vi "Tools VIs.vi"(6 "IMAQ Image Display Ref":refnum<vi>, 8 "Tool Name Text Ref":refnum<vi>, 9 "Left (Screen Coords, px)":i32=50, 11 "Top (Screen Coords, px)":i32=50) -> ()   [LabVIEW 2016]
uses:
  <vilib>/Utility/miscctls.llb/LVPointTypeDef.ctl
  <vilib>/Utility/miscctls.llb/LVRectTypeDef.ctl
  User32.dll
panel:
  in  "Show Cursor":bool=TRUE
  in  "Tools and ROI Menu":T1(radio)
  in  "Color Map Menu":T2(radio)
  in  "Scale All to This":bool
  in  "Load Image":bool
  in  "Tools and ROIs":bool
  in  "Lock Zoom and Pan Tools":bool
  in  "Pan Tool":bool
  in  "Reset Zoom":bool
  in  "Zoom Out":bool
  in  "Zoom In":bool
  in  "Auto Scale All":bool
  in  "Auto Scale":bool
  in  "Color Map":bool
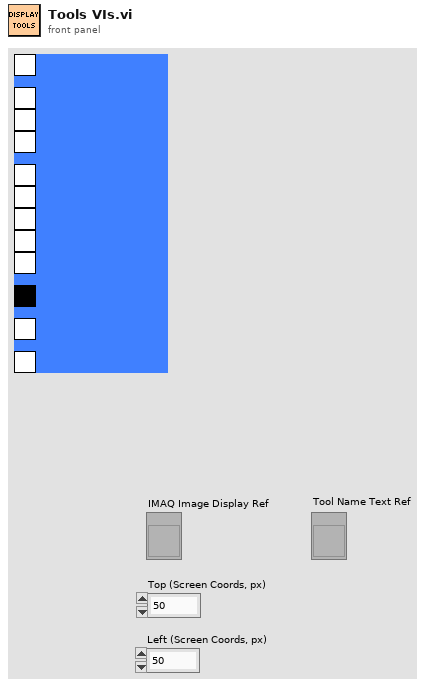
[diagram p1: front panel]
types:
  T1 = enum32{"Fitting Tool", "Merge Tool", "Smooth Tool", "Rectangular ROI", "Free Form ROI", "Clear ROI"}
  T2 = enum32{"Blue Z Scale", "Blue-White Z Scale", "Cyan Z Scale", "Fire Z Scale", "Glow Z Scale", "Green", "Green-White Z Scale", "Magenta Z Scale", "Red Z Scale", "Red-White Z Scale", "Yellow Z Scale"}
  T3 = enum32{"Invalid", "Standard", "Closed", "Hidden", "Minimized", "Maximized"}
  T4 = typedef "LVRectTypeDef.ctl" = cluster{"Left":i16, "Top":i16, "Right":i16, "Bottom":i16}
  T5 = typedef "LVPointTypeDef.ctl" = cluster{"Horizontal":i16, "Vertical":i16}
  T6 = enum16{"Always On", "Always Off", "Off While Running"}
  T7 = enum32{"Bad", "Idle", "Run top level", "Running"}
  T8 = typedef "lveventtype.ctl" = enum32{"Null", "Timeout", "Annotation Menu Selection", "Annotation Menu Selection?", "App Instance Close", "App Instance Close?", "Autoscale Range Change", "Bookmark Info Change", "Cell Edit", "Cell Edit?", "Cursor Grab", "Cursor Grab?", "Cursor Menu Selection", "Cursor Menu Selection?", "Cursor Move", "Cursor Release", "Data Change", "Direction Change", "Display State Change", "Drag Ended", "Drag Enter", "Drag Leave", "Drag Over", "Drag Source Update", "Drag Starting", "Drag Starting?", "Drop", "Exec State Change", "Key Down", "Key Down?", "Key Repeat", "Key Repeat?", "Key Up", "Listbox Double Click", "Menu Activation?", "Menu Selection (App)", "Menu Selection? (App)", "Menu Selection (User)", "Mouse Down", "Mouse Down?", "Mouse Enter", "Mouse Leave", "Mouse Move", "Mouse Up", "Mouse Wheel", "NI Security User Change (App)", "Pane Size", "Panel Close", "Panel Close?", "Panel Resize", "Plot Attribute Change", "Scale Range Change", "Shortcut Menu Activation?", "Shortcut Menu Selection (App)", "Shortcut Menu Selection? (App)", "Shortcut Menu Selection (User)", "Tree Double Click", "Tree Drag", "Tree Drag?", "Tree Drop", "Tree Drop?", "Tree Item Close", "Tree Item Close?", "Tree Item Open", "Tree Item Open?", "User Event", "Value Change"}
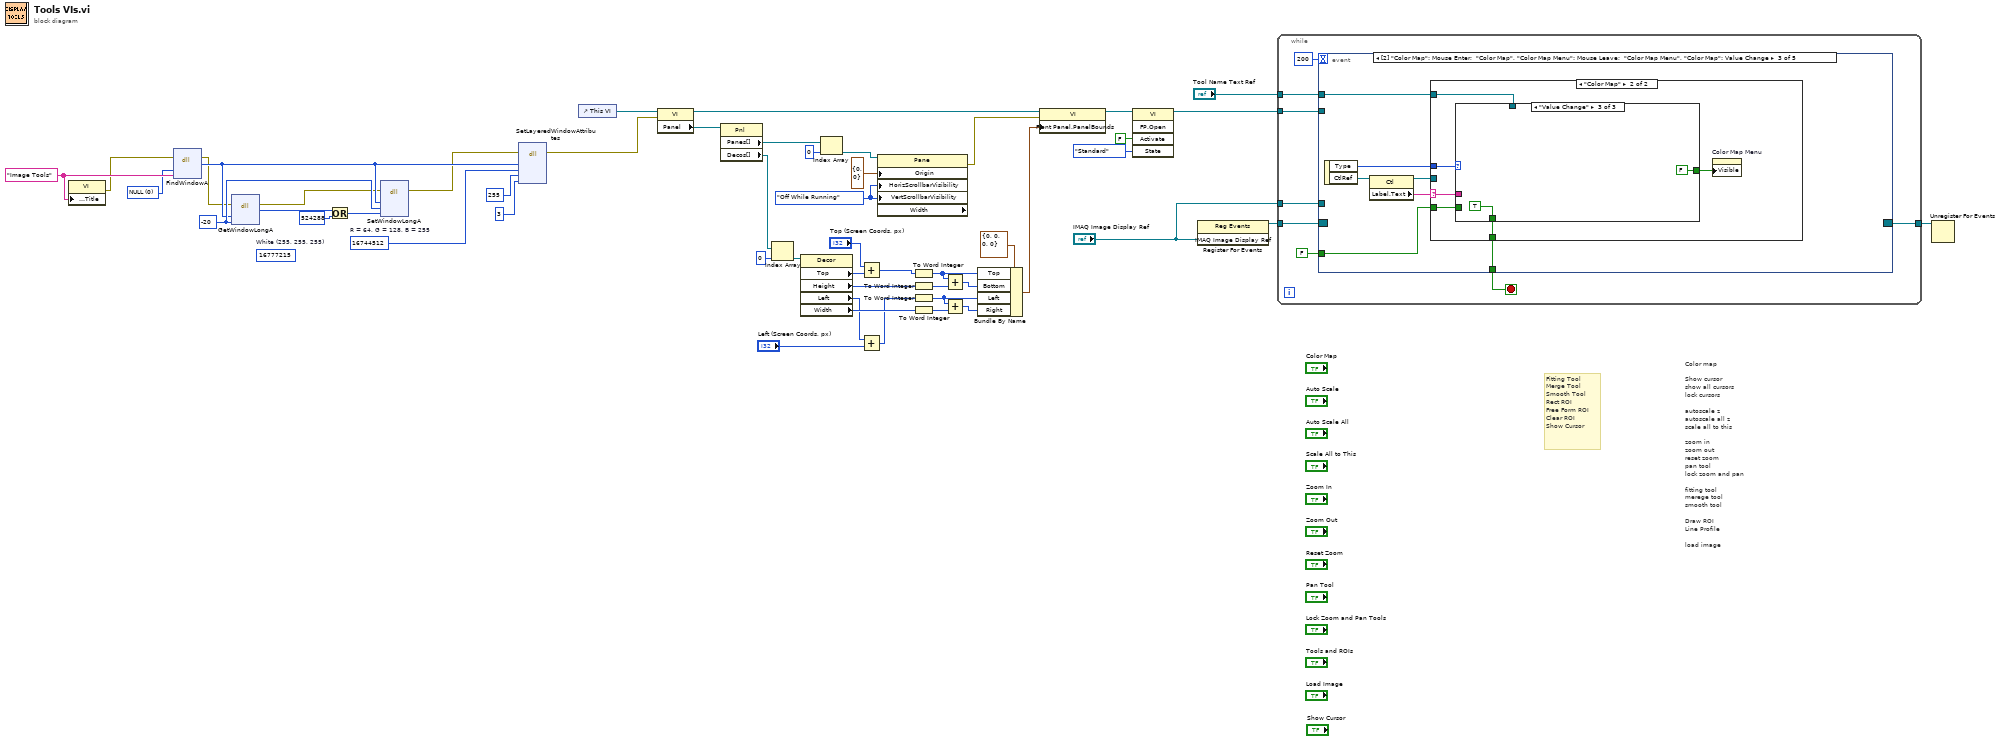
[diagram p0: block diagram]
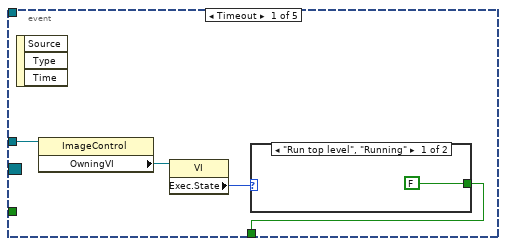
[diagram p2: hidden frame]
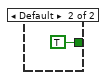
[diagram p3: hidden frame]
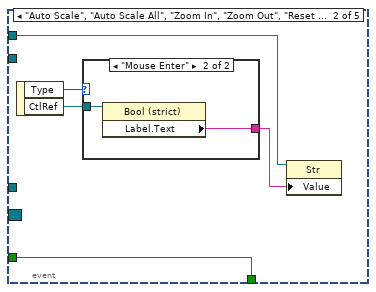
[diagram p4: hidden frame]
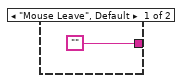
[diagram p5: hidden frame]
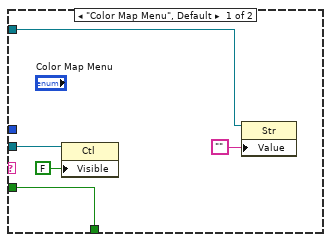
[diagram p6: hidden frame]
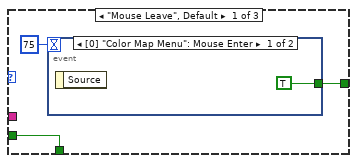
[diagram p7: hidden frame]
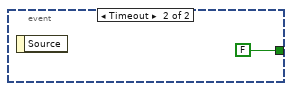
[diagram p8: hidden frame]
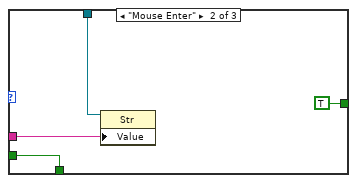
[diagram p9: hidden frame]
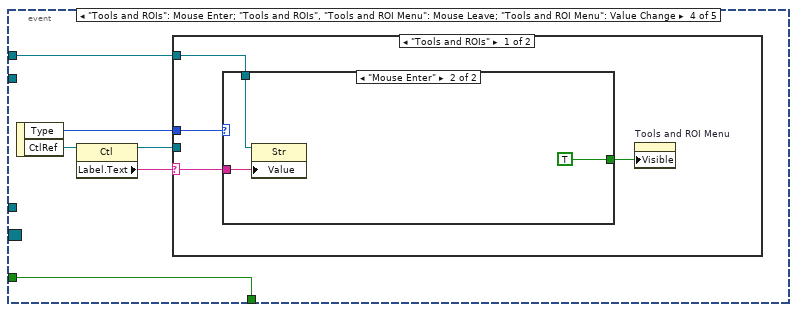
[diagram p10: hidden frame]
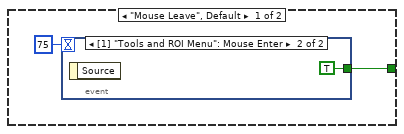
[diagram p11: hidden frame]
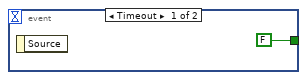
[diagram p12: hidden frame]
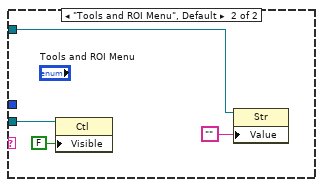
[diagram p13: hidden frame]
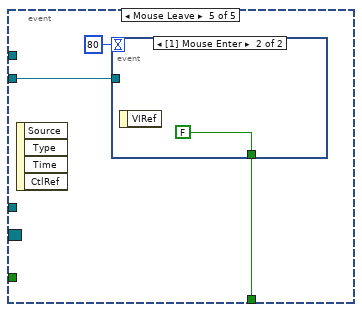
[diagram p14: hidden frame]
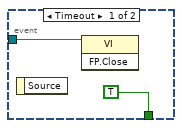
[diagram p15: hidden frame]
diagram:
  w11 = 16744512  # R = 64, G = 128, B = 255
  (unwired) 16777215  # White (255, 255, 255)
  w17 = 0 items=["NULL"]
  w21 = -20 ("nIndex")
  w23 = "Image Tools" ("Front Panel Window:Title")
  w47 = T6."Off While Running" ("Horizontal Scrollbar Visibility")
  # "Fitting Tool\nMerge Tool\nSmooth Tool\nRect ROI\nFree Form ROI\nClear ROI\nShow Cursor"
  # "Color map\n\nShow cursor\nshow all cursors\nlock cursors\n\nautoscale z\nautoscale all z\nscale all to this\n\nzoom in\nzoom out\nreset zoom\npan tool\nlock zoom and pan\n\nfitting tool\nmerege tool\nsmooth tool\n\nDraw ROI\nLine Profile\n\nload image"
  n1 = property class="VI"("Front Panel.Title"=w23) -> (error out=w10:errorcluster)  [unwired: 2 in, 1 out]
  n2 = dll-call lib="user32.dll" fn="FindWindowA" label="FindWindow"(error in=w10, "lpszClassName"=w17, "lpszWindowName"=w23) -> (error out=w14:errorcluster, "hWnd"=w20:i32)  [unwired: 3 in, 2 out]
  n3 = dll-call lib="USER32.DLL" fn="GetWindowLongA" label="getWindowLong"(error in=w14, "handle"=w20, "nIndex"=w21) -> (error out=w13:errorcluster, w19:i32)  [unwired: 4 in, 1 out]
  n4 = Or(x=w19, y=524288) -> (x .or. y?=w22:i32)
  n5 = dll-call lib="USER32.DLL" fn="SetWindowLongA" label="SetWindowLong"(error in=w13, "handle"=w20, "nIndex"=w21, "dwNewLong"=w22) -> (error out=w12:errorcluster)  [unwired: 5 in, 2 out]
  n6 = dll-call lib="USER32.DLL" fn="SetLayeredWindowAttributes" label="SetLayeredWindowAttributs"(error in=w12, "handle"=w20, "crkey"=w11, "bAlpha"=255, "dwFlags"=3) -> (error out=w9:errorcluster)  [unwired: 6 in, 2 out]
  n7 = control-ref of="This VI"() -> (w42:refnum<vi>)
  n8 = property class="VI"(reference=w42, error in=w9) -> (reference out=w41:refnum<vi>, "Panel"=w51:refnum<vi>)  [unwired: 1 out]
  n9 = property class="Pnl"(reference=w51) -> ("Panes[]"=w50:refnum<vi>[], "Decos[]"=w44:refnum<vi>[])  [unwired: 1 in, 2 out]
  n10 = Index Array(array=w44, index=0) -> (element=w43:refnum<vi>)
  n11 = property class="Decor"(reference=w43) -> ("Top"=w29:i32, "Height"=w39:u32, "Left"=w27:i32, "Width"=w35:u32)  [unwired: 1 in, 2 out]
  n12 = Index Array(array=w50, index=0) -> (element=w48:refnum<vi>)
  n13 = Add(x="Top (Screen Coords, px)", y=w29) -> (x+y=w28:i32)
  n14 = Add(x=w27, y="Left (Screen Coords, px)") -> (x+y=w26:i32)
  n15 = property class="Pane" props=["Origin", "HorizScrollbarVisibility", "VertScrollbarVisibility", "Width"](reference=w48, "Origin"=T5 {"Horizontal"=0, "Vertical"=0}, "HorizScrollbarVisibility"=w47, "VertScrollbarVisibility"=w47) -> (error out=w31:errorcluster)  [unwired: 1 in, 2 out]
  n16 = To Word Integer(number=w28) -> (16bit integer=w30:i16)
  n17 = To Word Integer(number=w39) -> (16bit integer=w38:i16)
  n18 = To Word Integer(number=w26) -> (16bit integer=w36:i16)
  n19 = To Word Integer(number=w35) -> (16bit integer=w34:i16)
  n20 = Add(x=w30, y=w38) -> (x+y=w37:i16)
  n21 = Add(x=w36, y=w34) -> (x+y=w33:i16)
  n22 = Bundle By Name(cluster=T4 {"Left"=0, "Top"=0, "Right"=0, "Bottom"=0} ("Front Panel Window:Panel Bounds"), "Top"=w30, "Bottom"=w37, "Left"=w36, "Right"=w33) -> (w32:T4)
  n23 = property class="VI"(reference=w41, error in=w31, "Front Panel.PanelBounds"=w32) -> (reference out=w6:refnum<vi>)  [unwired: 1 out]
  n24 = invoke class="VI" method="FP.Open"(reference=w6, "Activate"=FALSE ("Activate?"), "State"=T3."Standard") -> (reference out=w4:refnum<vi>)  [unwired: 2 in, 4 out]
  n25 = register-events("IMAQ Image Display Ref") -> (reference out=w5:refnum<event-registration>)  [unwired: 2 in, 1 out]
  n26 = while {
    tunnel: w5 -> [w57]
    tunnel: w4 -> [w56]
    tunnel: "IMAQ Image Display Ref" -> [w54]
    tunnel: "Tool Name Text Ref" -> [w53]
    tunnel: [w52] -> w1
    stop <- w59 stop-if-true
    n27 = event shown="[2] \"Color Map\": Mouse Enter;  \"Color Map\", \"Color Map Menu\": Mouse Leave;  \"Color Map Menu\", \"Color Map\": Value Change" {
      selector: w57 -> [_ _ _ _ _]
      dyn-events: [_ _ _ _ _] -> w52
      timeout: 200 -> [_ _ _ _ _]
      tunnel: [w60 w68 w76 w108 w124] -> w59
      tunnel: FALSE -> [_ w68 w75 w108 _]
      tunnel: w56 -> [_ _ _ _ w125]
      tunnel: w54 -> [w63 _ _ _ _]
      tunnel: w53 -> [_ w67 w74 w103 _]
      event Timeout {
        n28 = event-data() -> ()  [unwired: 1 in, 3 out]
        n29 = property class="ImageControl"(reference=w63) -> ("OwningVI"=w61:refnum<vi>)  [unwired: 1 in, 2 out]
        n30 = property class="VI"(reference=w61) -> ("Exec.State"=w62:T7)  [unwired: 1 in, 2 out]
        n31 = case shown="\"Run top level\", \"Running\"" w62 {
          tunnel: [FALSE TRUE] -> w60
          frame "Run top level", "Running" {
          }
          frame Default {
          }
        }
      }
      event "Auto Scale", "Auto Scale All", "Zoom In", "Zoom Out", "Reset Zoom", "Pan Tool", "Lock Zoom and Pan Tools", "Load Image", "Scale All to This", "Show Cursor": Mouse Enter; "Auto Scale", "Auto Scale All", "Zoom In", "Zoom Out", "Reset Zoom", "Pan Tool", "Lock Zoom and Pan Tools", "Load Image", "Scale All to This", "Show Cursor": Mouse Leave {
        n32 = event-data() -> ("Type"=w70:T8, "CtlRef"=w69:refnum<vi>)  [unwired: 1 in]
        n33 = case shown="\"Mouse Enter\"" w70 {
          tunnel: w69 -> [_ w73]
          tunnel: ["" w72] -> w66
          frame "Mouse Leave", Default {
          }
          frame "Mouse Enter" {
            n34 = property class="Bool (strict)"(reference=w73) -> ("Label.Text"=w72:string)  [unwired: 1 in, 2 out]
          }
        }
        n35 = property class="Str"(reference=w67, "Value"=w66) -> ()  [unwired: 1 in, 2 out]
      }
      event "Color Map": Mouse Enter; "Color Map", "Color Map Menu": Mouse Leave; "Color Map Menu", "Color Map": Value Change {
        n36 = event-data() -> ("Type"=w80:T8, "CtlRef"=w79:refnum<vi>)  [unwired: 1 in]
        n37 = property class="Ctl"(reference=w79) -> (reference out=w77:refnum<vi>, "Label.Text"=w78:string)  [unwired: 1 in, 1 out]
        n38 = case shown="\"Color Map\"" w78 {
          selector: w78 -> [_ w89]
          tunnel: w80 -> [_ w91]
          tunnel: w77 -> [w84 _]
          tunnel: [w83 w88] -> w76
          tunnel: w75 -> [w83 w87]
          tunnel: w74 -> [w82 w86]
          frame "Color Map Menu", Default {
            n39 = property class="Ctl"(reference=w84, "Visible"=FALSE) -> ()  [unwired: 1 in, 2 out]
            n40 = property class="Str"(reference=w82, "Value"="") -> ()  [unwired: 1 in, 2 out]
          }
          frame "Color Map" {
            n41 = case shown="\"Value Change\"" w91 {
              tunnel: [w93 TRUE ("Visible") FALSE ("Visible")] -> w90
              tunnel: w89 -> [_ w98 _]
              tunnel: [w92 w99 TRUE ("Visible")] -> w88
              tunnel: w87 -> [w92 w99 _]
              tunnel: w86 -> [_ w97 _]
              frame "Mouse Leave", Default {
                n42 = event shown="[0] \"Color Map Menu\": Mouse Enter" {
                  selector: _ -> [_ _]
                  dyn-events: _ -> [_ _]
                  timeout: 75 -> [_ _]
                  tunnel: [TRUE ("Visible") FALSE ("Visible")] -> w93
                  event "Color Map Menu": Mouse Enter {
                    n43 = event-data() -> ()  [unwired: 1 in, 1 out]
                  }
                  event Timeout {
                    n44 = event-data() -> ()  [unwired: 1 in, 1 out]
                  }
                }
              }
              frame "Mouse Enter" {
                n45 = property class="Str"(reference=w97, "Value"=w98) -> ()  [unwired: 1 in, 2 out]
              }
              frame "Value Change" {
              }
            }
            n46 = property on="Color Map Menu" class="RadioBtnsControl (strict)"("Visible"=w90) -> ()  [unwired: 2 in, 2 out]
          }
        }
      }
      event "Tools and ROIs": Mouse Enter; "Tools and ROIs", "Tools and ROI Menu": Mouse Leave; "Tools and ROI Menu": Value Change {
        n47 = event-data() -> ("Type"=w105:T8, "CtlRef"=w107:refnum<vi>)  [unwired: 1 in]
        n48 = property class="Ctl"(reference=w107) -> (reference out=w104:refnum<vi>, "Label.Text"=w106:string)  [unwired: 1 in, 1 out]
        n49 = case shown="\"Tools and ROIs\"" w106 {
          selector: w106 -> [w112 _]
          tunnel: w105 -> [w111 _]
          tunnel: w104 -> [_ w123]
          tunnel: w103 -> [w109 w120]
          frame "Tools and ROIs" {
            n50 = case shown="\"Mouse Enter\"" w111 {
              tunnel: w112 -> [_ w118]
              tunnel: [w113 TRUE] -> w110
              tunnel: w109 -> [_ w117]
              frame "Mouse Leave", Default {
                n51 = event shown="[1] \"Tools and ROI Menu\": Mouse Enter" {
                  selector: _ -> [_ _]
                  dyn-events: _ -> [_ _]
                  timeout: 75 -> [_ _]
                  tunnel: [FALSE TRUE] -> w113
                  event Timeout {
                    n52 = event-data() -> ()  [unwired: 1 in, 1 out]
                  }
                  event "Tools and ROI Menu": Mouse Enter {
                    n53 = event-data() -> ()  [unwired: 1 in, 1 out]
                  }
                }
              }
              frame "Mouse Enter" {
                n54 = property class="Str"(reference=w117, "Value"=w118) -> ()  [unwired: 1 in, 2 out]
              }
            }
            n55 = property on="Tools and ROI Menu" class="RadioBtnsControl (strict)"("Visible"=w110) -> ()  [unwired: 2 in, 2 out]
          }
          frame "Tools and ROI Menu", Default {
            n56 = property class="Ctl"(reference=w123, "Visible"=FALSE) -> ()  [unwired: 1 in, 2 out]
            n57 = property class="Str"(reference=w120, "Value"="") -> ()  [unwired: 1 in, 2 out]
          }
        }
      }
      event Mouse Leave {
        n58 = event-data() -> ()  [unwired: 1 in, 4 out]
        n59 = event shown="[1] Mouse Enter" {
          selector: _ -> [_ _]
          dyn-events: _ -> [_ _]
          timeout: 80 -> [_ _]
          tunnel: w125 -> [w127 _]
          tunnel: [TRUE FALSE] -> w124
          event Timeout {
            n60 = event-data() -> ()  [unwired: 1 in, 1 out]
            n61 = invoke class="VI" method="FP.Close"(reference=w127) -> ()  [unwired: 2 in, 3 out]
          }
          event Mouse Enter {
            n62 = event-data() -> ()  [unwired: 1 in, 1 out]
          }
        }
      }
    }
  }
  n63 = Unregister For Events(event registration refnum=w1) -> ()  [unwired: 1 in, 1 out]
